vi "listbox_selected_items.vi"(1 "Selected item number":i32[](array[numeric]), 2 "All items":string[](array[string])) -> (0 "Selected items":string[](array[string]))   [LabVIEW 2017]
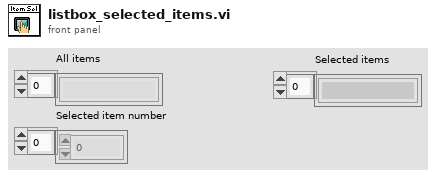
[diagram p1: front panel]
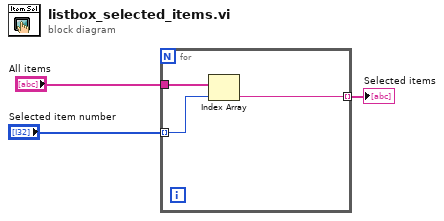
[diagram p0: block diagram]
diagram:
  n1 = for {
    tunnel: "All items" -> [w6]
    tunnel: "Selected item number" -> [w5] mode=indexing
    tunnel: [w4] -> w1 mode=indexing
    n2 = Index Array(array=w6, index=w5) -> (element=w4:string)
  }
  "Selected items" <- w1
